vi "LDA_analogue_start_time_sync_PN.vi"(4 "Window min. frac. size":dbl=0.01, 5 "BSA PM to TTL delay (s)":dbl=8e-06 format="%#_13g", 6 "Window reduction factor":dbl=0.707106781, 7 "Correlation peak fit method":enum32{"Max", "Quadratic", "Gaussian"}(ring)=enum."Quadratic", 8 "Pulse high threshold (V)":dbl=2.0, 9 "Analogue dt (s)":dbl, 10 "Analogue LDA burst pulse array (s)":dbl[](array[numeric]), 11 "LDA arrival times (s)":dbl[](array[numeric])) -> (0 "valid bursts array length check":bool, 3 "LDA start time rel. to Analogue (s)":dbl)   [LabVIEW 2016]
uses:
  <vilib>/Analysis/baseanly.llb/Normalize Vector.vi
  <vilib>/Analysis/2dsp.llb/1D Cross Correlation (DBL).vi
  <vilib>/Analysis/1siggen.llb/Ramp Pattern by Delta.vi
  <vilib>/Analysis/polynomials.llb/nth Derivative of Polynomial (DBL).vi
  <vilib>/Analysis/polynomials.llb/Polynomial Roots (DBL).vi
  <vilib>/Analysis/NI_AALPro.lvlib
  <vilib>/Analysis/NI_AALBase.lvlib
panel:
  out "Aligned burst times":T1(graph)
  out "Xcorr peak iterations":cluster{dbl[], dbl[]}(graph)
  out "Xcorr LDA timings":cluster{dbl[], "Best Gaussian Fit":dbl[]}[](graph)
  in  "Pts. either side of peak to use in fit":i32=3
  out "Analogue LDA burst pulse array":cluster{"index (row)":dbl, dbl, "Vout":dbl[]}(graph)
  out "Thresholded LDA burst times (valid only)":cluster{"index (row)":dbl, dbl, "Vout":dbl[]}(graph)
  out "Thresholded LDA arr time length":i32
  out "Thresholded LDA burst times (valid+invalid)":cluster{"index (row)":dbl, dbl, "Vout":dbl[]}(graph)
  out "LDA counted pulses (valid+invalid)":i32
  out "LDA arr_t length":i32
  # "equal length?"
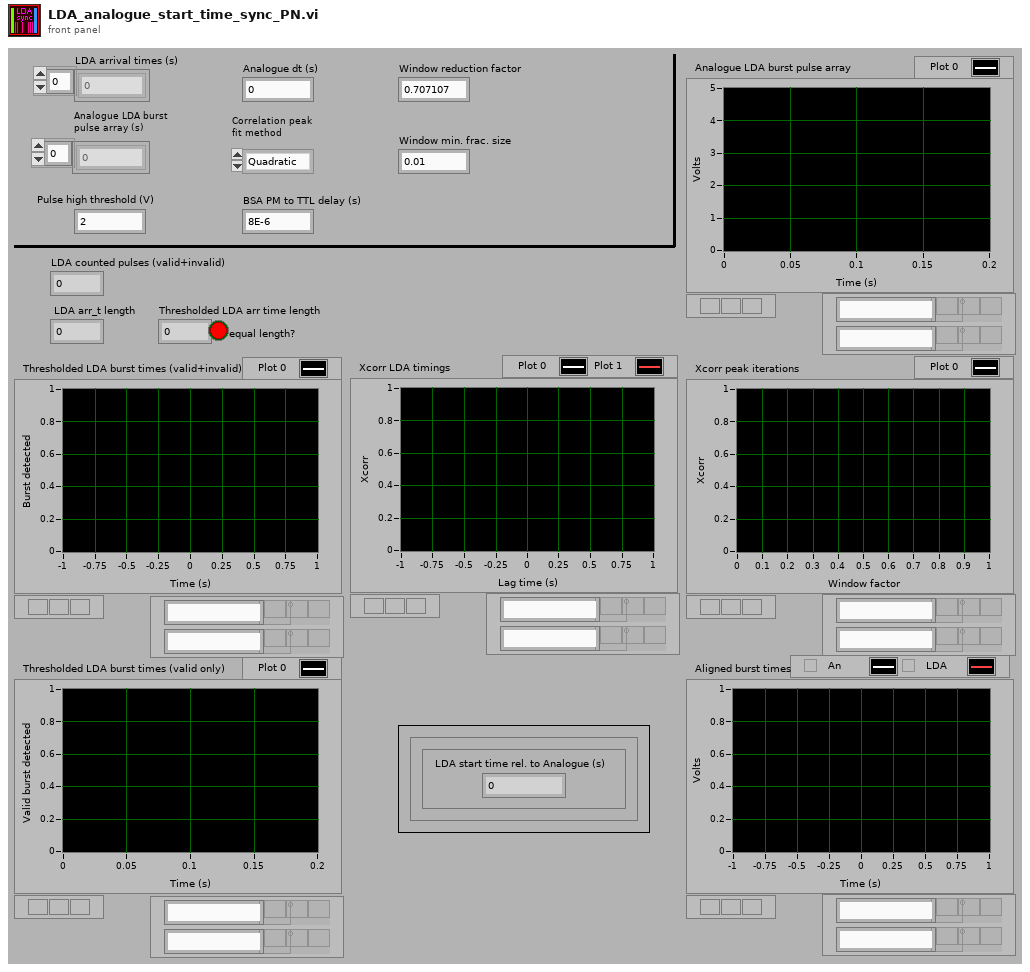
[diagram p1: front panel]
types:
  T1 = cluster{"index (row)":dbl, "Analogue dt (s)":dbl, "Vout":dbl[]}[]
  T2 = cluster{"index (row)":dbl, "Analogue dt (s)":dbl, "Vout":dbl[]}
  T3 = cluster{"index (row)":dbl, "Analogue dt (s)":dbl, "Analogue LDA burst pulse array (s)":dbl[]}
  T4 = cluster{"center":dbl, "Analogue dt (s)":dbl, "Vout":dbl[]}
  T5 = cluster{"Ramp Pattern":dbl[], "Best Gaussian Fit":dbl[]}[]
  T6 = cluster{"center":dbl, "Analogue dt (s)":dbl, "Vout":dbl[]}[]
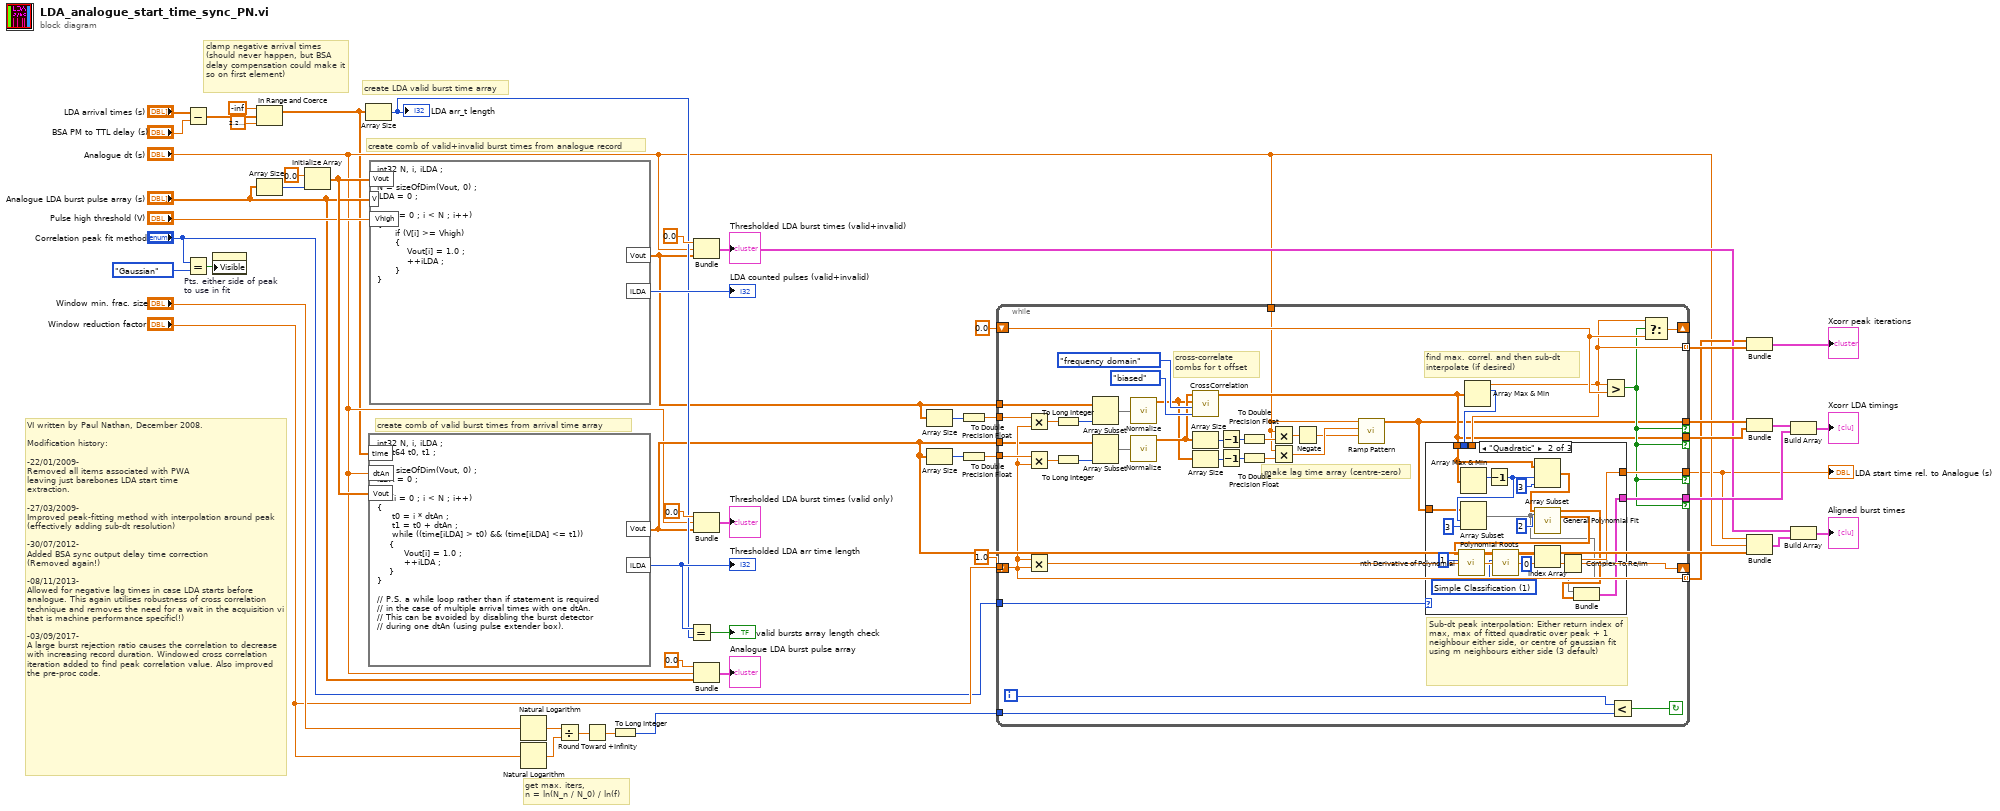
[diagram p0: block diagram]
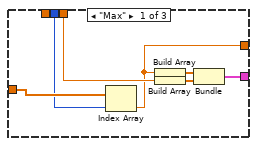
[diagram p2: hidden frame]
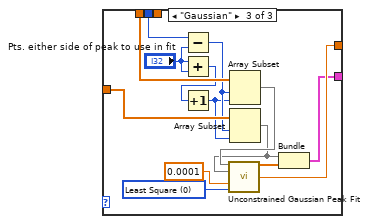
[diagram p3: hidden frame]
diagram:
  # "clamp negative arrival times (should never happen, but BSA delay compensation could make it so on first element)"
  # "get max. iters,\nn = ln(N_n / N_0) / ln(f)"
  # "create LDA valid burst time array"
  # "VI written by Paul Nathan, December 2008.\n\nModification history:\n\n-22/01/2009-\nRemoved all items associated with PWA\nleaving just barebones LDA start time\nextraction.\n\n-27/03/2009-\nImproved peak-fitting method with interpolation around peak (effectively adding sub-dt resolution)\n\n-30/07/2012-\nAdded BSA sync output delay time correction\n(Removed again!)\n\n-08/11/2013-\nAllowed for negative lag times in case LDA starts before analogue. This again utilises robustness of cross correlation technique and removes the need for a wait in the acquisition vi that is machine performance specific(!)\n\n-03/09/2017-\nA large burst rejection ratio causes the correlation to decrease with increasing record duration. Windowed cross correlation iteration added to find peak correlation value. Also improved the pre-proc code."
  # "create comb of valid+invalid burst times from analogue record"
  # "create comb of valid burst times from arrival time array"
  n1 = Subtract(x="LDA arrival times (s)", y="BSA PM to TTL delay (s)") -> (x-y=w4:dbl[])
  n2 = Equal?(x="Correlation peak fit method", y=enum32{"Max", "Quadratic", "Gaussian"}."Gaussian") -> (x = y?=w37:bool)
  n3 = property on="Pts. either side of peak to use in fit" class="DigNum (strict)"("Visible"=w37) -> ()  [unwired: 2 in, 2 out]
  n4 = In Range and Coerce(upper limit=-inf, x=w4, lower limit=2.220446049250313e-16) -> (coerced(x)=w1:dbl[])  [unwired: 1 out]
  n5 = Array Size(array="Analogue LDA burst pulse array (s)") -> (size(s)=w47:i32)
  n6 = Initialize Array(0.0 ("element"), w47) -> (w46:dbl[])
  n7 = Array Size(array=w1) -> (size(s)=w32:i32)
  "LDA arr_t length" <- w32
  n8 = formula code="int32 N, i, iLDA ;\nfloat64 t0, t1 ;\n\nN = sizeOfDim(Vout, 0) ;\niLDA = 0 ;\n\nfor (i = 0 ; i < N ; i++)\n{\n     t0 = i * dtAn ;\n     t1 = t0 + dtAn ;\n     while ((time[iLDA] > t0) && (time[iLDA] <= t1)) \n    {  \n         Vout[i] = 1.0 ;\n         ++iLDA ;\n    }\n}\n\n// P.S. a while loop rather than if statement is required\n// in the case of multiple arrival times with one dtAn.\n// This can be avoided by disabling the burst detector\n// during one dtAn (using pulse extender box)."("dtAn"="Analogue dt (s)", "time"=w1, "Vout"=w46) -> ("Vout"=w17:dbl[], "iLDA"=w33:i32)
  "Thresholded LDA arr time length" <- w33
  n9 = formula code="int32 N, i, iLDA ;\n\nN = sizeOfDim(Vout, 0) ;\niLDA = 0 ;\n\nfor (i = 0 ; i < N ; i++)\n{\n      if (V[i] >= Vhigh)\n      {\n          Vout[i] = 1.0 ;\n          ++iLDA ;\n      }\n}"("V"="Analogue LDA burst pulse array (s)", "Vhigh"="Pulse high threshold (V)", "Vout"=w46) -> ("Vout"=w21:dbl[], "iLDA"=→"LDA counted pulses (valid+invalid)":i32)
  n10 = Natural Logarithm(1:"Window min. frac. size") -> (0:w28:dbl)
  n11 = Natural Logarithm(1:"Window reduction factor") -> (0:w27:dbl)
  n12 = Divide(x=w28, y=w27) -> (x/y=w26:dbl)
  n13 = Round Toward +Infinity(x=w26) -> (ceil(x): smallest int >= x=w25:dbl)
  n14 = To Long Integer(number=w25) -> (32bit integer=w24:i32)
  n15 = Equal?(x=w33, y=w32) -> (x = y?=→"valid bursts array length check":bool)
  n16 = Bundle("index (row)"=0.0, "Analogue dt (s)"="Analogue dt (s)", "Vout"=w21) -> (w19:T2)  [unwired: 1 out]
  "Thresholded LDA burst times (valid+invalid)" <- w19
  n17 = Bundle("index (row)"=0.0, "Analogue dt (s)"="Analogue dt (s)", "Vout"=w17) -> (→"Thresholded LDA burst times (valid only)":T2)  [unwired: 1 out]
  n18 = Bundle("index (row)"=0.0, "Analogue dt (s)"="Analogue dt (s)", "Analogue LDA burst pulse array (s)"="Analogue LDA burst pulse array (s)") -> (→"Analogue LDA burst pulse array":T3)  [unwired: 1 out]
  n19 = Array Size(array=w21) -> (size(s)=w15:i32)
  n20 = Array Size(array=w17) -> (size(s)=w14:i32)
  n21 = To Double Precision Float(number=w15) -> (double precision float=w12:dbl)
  n22 = To Double Precision Float(number=w14) -> (double precision float=w13:dbl)
  n23 = while {
    tunnel: "Analogue dt (s)" -> [w57]
    tunnel: [w88] -> w39 if=w76
    tunnel: "Correlation peak fit method" -> [w87]
    tunnel: [w86] -> w7 if=w76
    tunnel: [w53] -> w36 if=w76
    tunnel: [w68] -> w35 if=w76
    tunnel: w21 -> [w55]
    tunnel: w17 -> [w54]
    shift-right: [w81] -> _
    shift-left: 0.0 -> [w80]
    tunnel: [w79] -> w30 mode=indexing
    tunnel: w24 -> [w78]
    tunnel: [w69] -> w16 mode=indexing
    shift-right: [w70] -> _
    shift-left: 1.0 ("start") -> [w69]
    tunnel: w12 -> [w73]
    tunnel: w13 -> [w74]
    tunnel: "Window reduction factor" -> [w75]
    i -> [w77]
    stop <- w52 continue-if-true
    # "make lag time array (centre-zero)"
    # "find max. correl. and then sub-dt interpolate (if desired)"
    # "Sub-dt peak interpolation: Either return index of max, max of fitted quadratic over peak + 1 neighbour either side, or centre of gaussian fit using m neighbours either side (3 default)"
    # "cross-correlate combs for t offset"
    n24 = Multiply(x=w73, y=w69) -> (x*y=w82:dbl)
    n25 = Multiply(x=w74, y=w69) -> (x*y=w83:dbl)
    n26 = Multiply(x=w69, y=w75) -> (x*y=w70:dbl)
    n27 = To Long Integer(number=w82) -> (32bit integer=w71:i32)
    n28 = To Long Integer(number=w83) -> (32bit integer=w72:i32)
    n29 = Array Subset(array=w55, length=w71) -> (w85:dbl[])  [unwired: 1 in]
    n30 = Array Subset(array=w54, length=w72) -> (w84:dbl[])  [unwired: 1 in]
    n31 = call-poly <vilib>:"Normalize.vi"("Vector"=w85) -> ("Normalized Vector"=w62:dbl[])  [unwired: 1 in, 3 out]
    n32 = call-poly <vilib>:"Normalize.vi"("Vector"=w84) -> ("Normalized Vector"=w66:dbl[])  [unwired: 1 in, 3 out]
    n33 = call-poly <vilib>:"CrossCorrelation.vi"("normalization"=enum32{"none", "unbiased", "biased"}."biased", "algorithm"=enum32{"direct", "frequency domain"}."frequency domain", "Y"=w62, "X"=w66) -> ("Rxy"=w68:dbl[])  [unwired: 7 out]
    n34 = Array Size(array=w66) -> (size(s)=w61:i32)
    n35 = Array Size(array=w62) -> (size(s)=w60:i32)
    n36 = Decrement(x=w61) -> (x-1=w59:i32)
    n37 = Decrement(x=w60) -> (x-1=w58:i32)
    n38 = To Double Precision Float(number=w59) -> (double precision float=w65:dbl)
    n39 = To Double Precision Float(number=w58) -> (double precision float=w56:dbl)
    n40 = Multiply(x=w57, y=w65) -> (x*y=w64:dbl)
    n41 = Multiply(x=w57, y=w56) -> (x*y=w67:dbl)
    n42 = Negate(x=w64) -> (-x=w63:dbl)
    n43 = call-poly <vilib>:"Ramp Pattern.vi"("start"=w63, "end"=w67, "delta"=w57) -> ("Ramp Pattern"=w53:dbl[])  [unwired: 6 in, 2 out]
    n44 = Array Max & Min(array=w68) -> (max value=w79:dbl, max index (indices)=w89:i32)  [unwired: 2 out]
    n45 = case shown="\"Quadratic\"" w87 {
      tunnel: w68 -> [_ w106 w128]
      tunnel: [w93 w107 w130] -> w86
      tunnel: [w98 w104 w120] -> w88
      tunnel: w53 -> [w94 w100 w125]
      tunnel: w89 -> [w92 _ w127]
      tunnel: w79 -> [w95 _ _]
      frame "Max" {
        n46 = Index Array(array=w94, index=w92) -> (element=w93:dbl)
        n47 = Build Array(w93) -> (w96:dbl[])
        n48 = Build Array(w95) -> (w97:dbl[])
        n49 = Bundle(w96, w97) -> (w98:cluster{dbl[], dbl[]})  [unwired: 1 out]
      }
      frame "Quadratic" {
        w111 = u16 1 items=["General", "Simple Classification", "Refinement", "Advanced Refinement"] ("option")
        n50 = Array Max & Min(array=w106) -> (max index (indices)=w116:i32)  [unwired: 3 out]
        n51 = Decrement(x=w116) -> (x-1=w101:i32)
        n52 = Array Subset(array=w100, index=w101, length=3) -> (w99:dbl[])
        n53 = Array Subset(array=w106, index=w101, length=3) -> (w115:dbl[])
        n54 = call <vilib>:"General Polynomial Fit.vi"("Y"=w115, "polynomial order"=2, "X"=w99) -> ("Best Polynomial Fit"=w103:dbl[], "Polynomial Coefficients"=w105:dbl[])  [unwired: 9 in, 2 out]
        n55 = call-poly <vilib>:"nth Derivative of Polynomial.vi"("order"=1, "P(x)"=w105) -> ("Nth Derivative of P(x)"=w112:dbl[])  [unwired: 9 out]
        n56 = call-poly <vilib>:"Polynomial Roots.vi"("option"=w111, "P(x)"=w112) -> ("Roots"=w110:cdb[])  [unwired: 9 out]
        n57 = Index Array(array=w110, index=0) -> (element=w108:cdb)
        n58 = Complex To Re/Im(x + iy=w108) -> (x=w107:dbl)  [unwired: 1 out]
        n59 = Bundle(w99, "Best Polynomial Fit"=w103) -> (w104:cluster{dbl[], "Best Polynomial Fit":dbl[]})  [unwired: 1 out]
      }
      frame "Gaussian" {
        w129 = u16 0 items=["Least Square", "Least Absolute Residual", "Bisquare"] ("method")
        n60 = Subtract(x=w127, y="Pts. either side of peak to use in fit") -> (x-y=w124:i32)
        n61 = Add(x="Pts. either side of peak to use in fit", y="Pts. either side of peak to use in fit") -> (x+y=w118:i32)
        n62 = Increment(x=w118) -> (x+1=w119:i32)
        n63 = Array Subset(array=w128, index=w124, length=w119) -> (w123:dbl[])
        n64 = Array Subset(array=w125, index=w124, length=w119) -> (w121:dbl[])
        n65 = call <vilib>:"Unconstrained Gaussian Peak Fit.vi"("Y"=w123, "X"=w121, "tolerance"=0.0001, "method"=w129) -> ("Best Gaussian Fit"=w122:dbl[], "center"=w130:dbl)  [unwired: 6 in, 4 out]
        n66 = Bundle(w121, "Best Gaussian Fit"=w122) -> (w120:cluster{dbl[], "Best Gaussian Fit":dbl[]})  [unwired: 1 out]
      }
    }
    n67 = Greater?(x=w79, y=w80) -> (0:w76:bool)
    n68 = Less?(x=w77, y=w78) -> (x < y?=w52:bool)
    n69 = Select(t=w79, s=w76, f=w80) -> (s? t:f=w81:dbl)
  }
  "LDA start time rel. to Analogue (s)" <- w7
  n70 = Bundle(w16, w30) -> (→"Xcorr peak iterations":cluster{dbl[], dbl[]})  [unwired: 1 out]
  n71 = Bundle("Ramp Pattern"=w36, "Rxy"=w35) -> (w22:cluster{"Ramp Pattern":dbl[], "Rxy":dbl[]})  [unwired: 1 out]
  n72 = Bundle("center"=w7, "Analogue dt (s)"="Analogue dt (s)", "Vout"=w17) -> (w18:T4)  [unwired: 1 out]
  n73 = Build Array(w22, w39) -> (→"Xcorr LDA timings":T5)
  n74 = Build Array(w19, w18) -> (→"Aligned burst times":T6)
